vi "AIT 664 - Add End System.vi"(0 "Node Ptr":u64 format="%.0x", 5 "664 End System":T1, 11 "error in (no error)":errorcluster) -> (6 "Section Ptr Out":T8 format="%.0x", 15 "error out":errorcluster)   [LabVIEW 2013, in "AIT 664 Custom Device.lvlib"]
doc: "Add an end system to the device tree."
uses:
  AIT 664 Custom Device.lvlib
  <vilib>/NI Veristand/Custom Device API/Custom Device Item Ref.ctl
  Controls/664 - XML End System Description.ctl
  Controls/664 - XML Output VL.ctl
  Controls/664 - XML Tx Message Port.ctl
  Controls/664 - Sampling Type.ctl
  Controls/664 -Param.ctl
  Controls/664 - XML Input VL.ctl
  Controls/664 - XML Rx Message Port.ctl
  Controls and Global/Global.vi
  <vilib>/NI Veristand/Custom Device API/Set Item Property (String).vi
  <vilib>/NI Veristand/Custom Device API/Set Item Property (U32).vi
  <vilib>/NI Veristand/Custom Device API/Custom Device API.lvlib
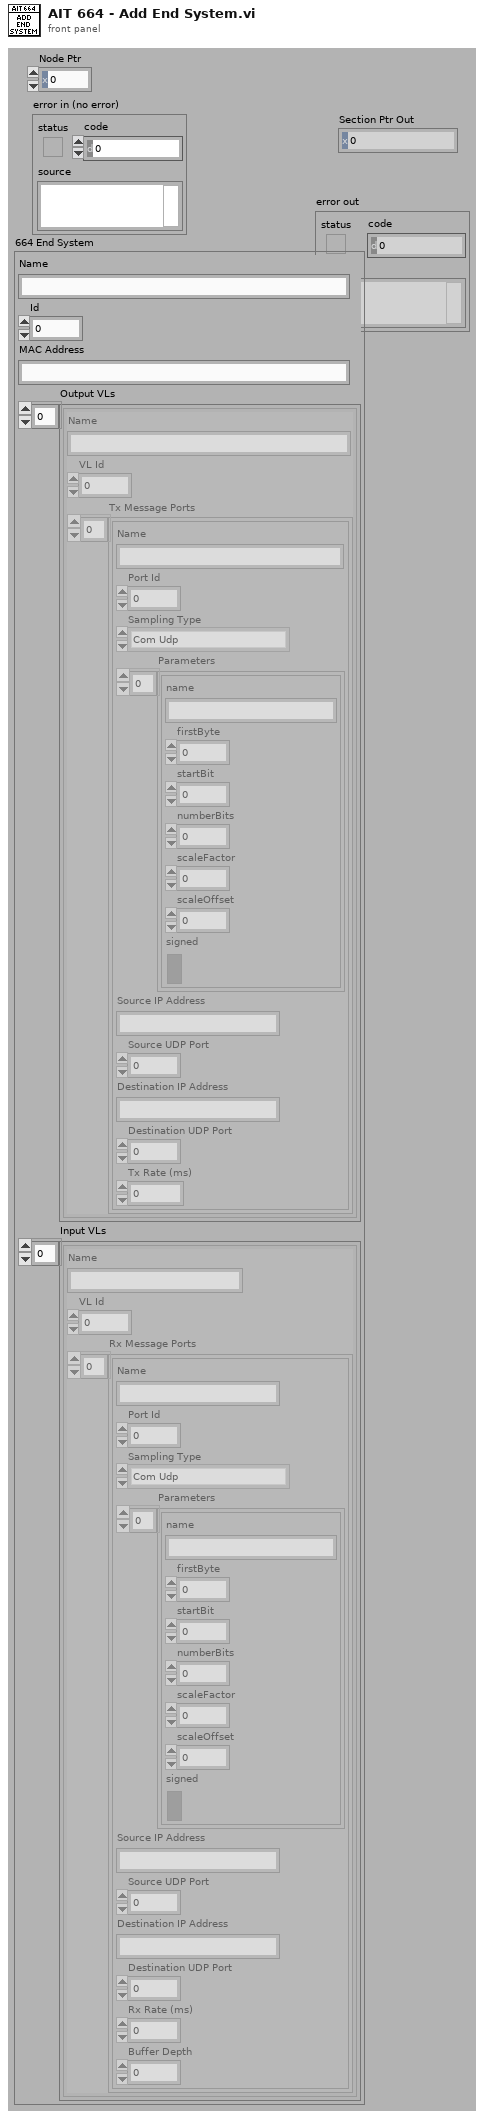
[diagram p1: front panel]
types:
  T1 = typedef "AIT 664 Custom Device.lvlib/664 - XML End System Description.ctl" = cluster{"Name":string, "Id":u32, "MAC Address":string, "Output VLs":T2[], "Input VLs":T6[]}
  T2 = typedef "AIT 664 Custom Device.lvlib/664 - XML Output VL.ctl" = cluster{"Name":string, "VL Id":u32, "Tx Message Ports":T3[]}
  T3 = typedef "AIT 664 Custom Device.lvlib/664 - XML Tx Message Port.ctl" = cluster{"Name":string, "Port Id":u32, "Sampling Type":T4, "Parameters":T5[], "Source IP Address":string, "Source UDP Port":u32, "Destination IP Address":string, "Destination UDP Port":u32, "Tx Rate (ms)":u32}
  T4 = typedef "AIT 664 Custom Device.lvlib/664 - Sampling Type.ctl" = enum16{"Com Udp", "Com Udp Queuing", "Sap Udp", "Sap Ip", "Sap Mac", "Unknown"}
  T5 = typedef "AIT 664 Custom Device.lvlib/664 -Param.ctl" = cluster{"name":string, "firstByte":i32, "startBit":i32, "numberBits":i32, "scaleFactor":dbl, "scaleOffset":dbl, "signed":bool}
  T6 = typedef "AIT 664 Custom Device.lvlib/664 - XML Input VL.ctl" = cluster{"Name":string, "VL Id":u32, "Rx Message Ports":T7[]}
  T7 = typedef "AIT 664 Custom Device.lvlib/664 - XML Rx Message Port.ctl" = cluster{"Name":string, "Port Id":u32, "Sampling Type":T4, "Parameters":T5[], "Source IP Address":string, "Source UDP Port":u32, "Destination IP Address":string, "Destination UDP Port":u32, "Rx Rate (ms)":u32, "Buffer Depth":u32}
  T8 = typedef "Custom Device API.lvlib/Custom Device Item Ref.ctl" = u64
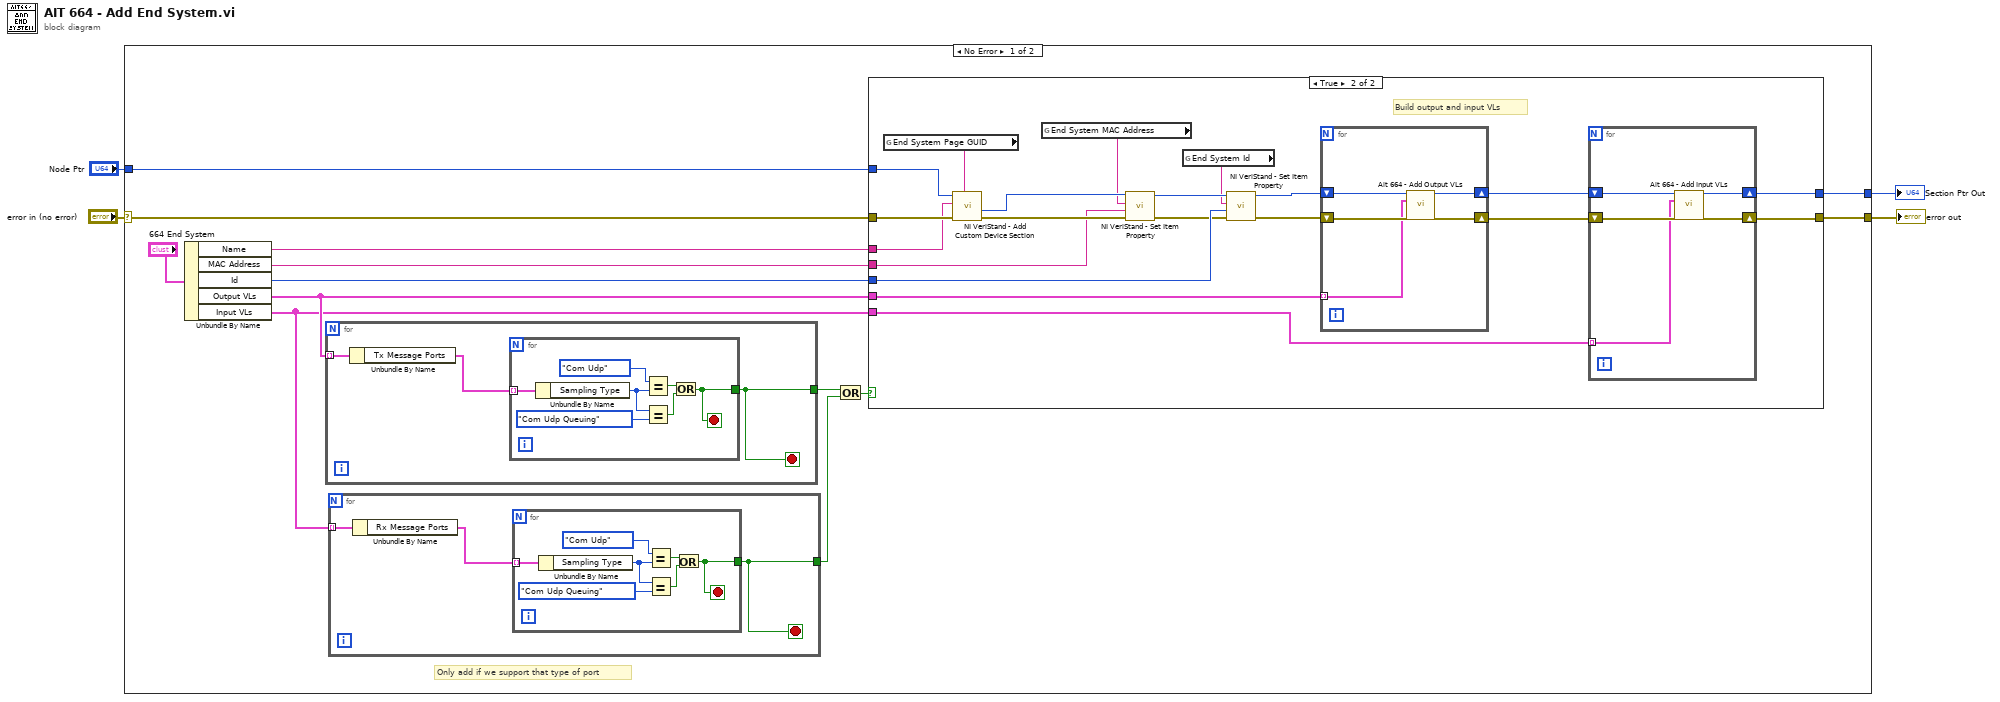
[diagram p0: block diagram]
diagram:
  n1 = case shown="No Error" "error in (no error)" {
    selector: "error in (no error)" -> [w16 w69]
    tunnel: "Node Ptr" -> [w17 _]
    tunnel: [w15 w69] -> w2
    tunnel: [w14 _] -> w1
    frame No Error {
      # "Only add if we support that type of port"
      n2 = Unbundle By Name("664 End System") -> ("Name"=w12:string, "MAC Address"=w11:string, "Id"=w10:u32, "Output VLs"=w6:T2[], "Input VLs"=w5:T6[])
      n3 = for {
        tunnel: w6 -> [w61] mode=indexing
        tunnel: [w59] -> w9
        stop <- w59 stop-if-true
        n4 = Unbundle By Name(w61) -> ("Tx Message Ports"=w60:T3[])
        n5 = for {
          tunnel: w60 -> [w68] mode=indexing
          tunnel: [w62] -> w59
          stop <- w62 stop-if-true
          n6 = Unbundle By Name(w68) -> ("Sampling Type"=w66:T4)
          n7 = Equal?(x=664_-_Sampling_Type."Com Udp" ("Sampling Type"), y=w66) -> (x = y?=w64:bool)
          n8 = Equal?(x=w66, y=664_-_Sampling_Type."Com Udp Queuing" ("Sampling Type")) -> (x = y?=w63:bool)
          n9 = Or(x=w64, y=w63) -> (x .or. y?=w62:bool)
        }
      }
      n10 = for {
        tunnel: w5 -> [w51] mode=indexing
        tunnel: [w49] -> w8
        stop <- w49 stop-if-true
        n11 = Unbundle By Name(w51) -> ("Rx Message Ports"=w50:T7[])
        n12 = for {
          tunnel: w50 -> [w58] mode=indexing
          tunnel: [w52] -> w49
          stop <- w52 stop-if-true
          n13 = Unbundle By Name(w58) -> ("Sampling Type"=w56:T4)
          n14 = Equal?(x=664_-_Sampling_Type."Com Udp" ("Sampling Type"), y=w56) -> (x = y?=w54:bool)
          n15 = Equal?(x=w56, y=664_-_Sampling_Type."Com Udp Queuing" ("Sampling Type")) -> (x = y?=w53:bool)
          n16 = Or(x=w54, y=w53) -> (x .or. y?=w52:bool)
        }
      }
      n17 = Or(x=w9, y=w8) -> (x .or. y?=w7:bool)
      n18 = case shown="True" w7 {
        tunnel: w17 -> [_ w38]
        tunnel: w16 -> [w18 w37]
        tunnel: [w18 w36] -> w15
        tunnel: [_ w19] -> w14
        tunnel: w12 -> [_ w31]
        tunnel: w11 -> [_ w30]
        tunnel: w10 -> [_ w29]
        tunnel: w6 -> [_ w28]
        tunnel: w5 -> [_ w27]
        frame False {
        }
        frame True {
          # "Build output and input VLs"
          n19 = global read "Global.vi" "End System Page GUID"() -> (w33:string)
          n20 = call <vilib>:"NI VeriStand - Add Custom Device Section.vi"("GUID (Default Section)"=w33, "error in (no error)"=w37, "Section Name"=w31, "Parent Ref in"=w38) -> ("error out"=w35:errorcluster, "Section Ptr"=w34:T8)  [unwired: 4 in, 2 out]
          n21 = global read "Global.vi" "End System MAC Address"() -> (w26:string)
          n22 = call-poly <vilib>:"NI VeriStand - Set Item Property.vi"("error in (no error)"=w35, "Value"=w30, "Property Name"=w26, "Item Ref in"=w34) -> ("error out"=w25:errorcluster, "Item Ref out"=w24:T8)  [unwired: 5 in, 1 out]
          n23 = global read "Global.vi" "End System Id"() -> (w23:string)
          n24 = call-poly <vilib>:"NI VeriStand - Set Item Property.vi"("error in (no error)"=w25, "Value"=w29, "Property Name"=w23, "Item Ref in"=w24) -> ("error out"=w22:errorcluster, "Item Ref out"=w32:T8)  [unwired: 5 in, 1 out]
          n25 = for {
            tunnel: w28 -> [w46] mode=indexing
            shift-right: [w45] -> w21
            shift-left: w22 -> [w48]
            shift-right: [w44] -> w20
            shift-left: w32 -> [w47]
            n26 = call "Ait 664 - Add Output VLs.vi"("Item Ref in"=w47, "Output VL"=w46, "error in (no error)"=w48) -> ("Item Ref out"=w44:T8, "error out"=w45:errorcluster)  [unwired: 11 in]
          }
          n27 = for {
            shift-right: [w41] -> w36
            shift-left: w21 -> [w43]
            tunnel: w27 -> [w40] mode=indexing
            shift-right: [w39] -> w19
            shift-left: w20 -> [w42]
            n28 = call "Ait 664 - Add Input VLs.vi"("Item Ref in"=w42, "Input VL"=w40, "error in (no error)"=w43) -> ("Item Ref out"=w39:T8, "error out"=w41:errorcluster)  [unwired: 11 in]
          }
        }
      }
    }
    frame Error {
    }
  }
  "error out" <- w2
  "Section Ptr Out" <- w1
